vi "Update Table Row Text Color.vi"(7 "Table row count":i32, 10 "Channel count":i32, 11 "Table":refnum<vi>) -> ()   [LabVIEW 2021]
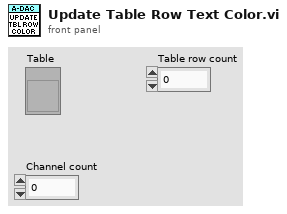
[diagram p1: front panel]
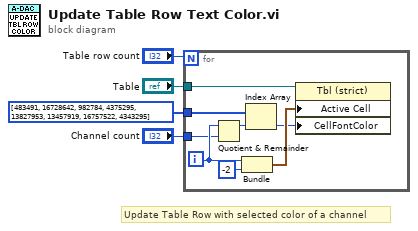
[diagram p0: block diagram]
diagram:
  # "Update Table Row with selected color of a channel"
  n1 = for {
    N: "Table row count" -> [_]
    tunnel: "Channel count" -> [w6]
    tunnel: "Table" -> [w12]
    tunnel: u32[] [483491, 16728642, 982784, 4375295, 13827953, 13457919, 16757522, 4343295] -> [w9]
    i -> [w7]
    n2 = Quotient & Remainder(x=w7, y=w6) -> (x-y*floor(x/y)=w5:i32)  [unwired: 1 out]
    n3 = Bundle(w7, -2) -> (w10:cluster{i32, i32})  [unwired: 1 in]
    n4 = Index Array(array=w9, index=w5) -> (element=w8:u32)
    n5 = property class="Tbl (strict)"(reference=w12, "Active Cell"=w10, "CellFontColor"=w8) -> ()  [unwired: 1 in, 2 out]
  }
